vi "DeQ Helper Loop Q DVR.vi"(10 "Helper Loop Q DVR":refnum<data-value>) -> (0 "error out":errorcluster, 2 "Helper Loop":refnum<class "Helper Loop.lvclass">)   [LabVIEW 2021, in "Helper Loop.lvclass"]
uses:
  Helper Loop.lvclass
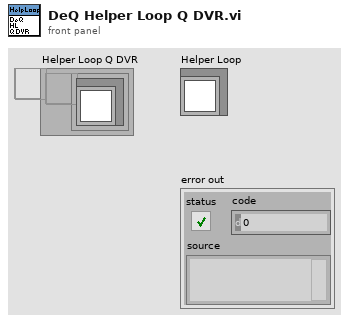
[diagram p1: front panel]
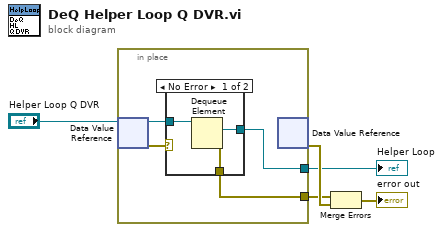
[diagram p0: block diagram]
diagram:
  n1 = in-place {
    in-place-border: [w8] -> w4
    in-place-border: [w7] -> w1
    n2 = in-place-dvr #1("Helper Loop Q DVR") -> (w9:refnum<queue>, w6:errorcluster)
    n3 = case shown="No Error" w6 {
      selector: w6 -> [_ w13]
      tunnel: w9 -> [w12 _]
      tunnel: [w11 w13] -> w8
      tunnel: [w10 _] -> w7
      frame No Error {
        n4 = Dequeue Element(queue=w12) -> (element=w10:refnum<class "Helper Loop.lvclass">, error out=w11:errorcluster)  [unwired: 2 in, 2 out]
      }
      frame Error {
      }
    }
    n5 = in-place-dvr #1() -> (w5:errorcluster)  [unwired: 1 in, 1 out]
  }
  "Helper Loop" <- w1
  n6 = Merge Errors(w4, w5) -> (→"error out":errorcluster)
